vi "new.vi"(8 "error in (no error)":errorcluster, 11 "description":string) -> (0 "error out":errorcluster, 3 "ExampleTask_StopNotifier out":refnum<class "Task_BoolStopNotifier.lvclass">)   [LabVIEW 2023, in "Task_BoolStopNotifier.lvclass"]
doc: "Constructor"
uses:
  Task_BoolStopNotifier.lvclass
  Task_BoolStopNotifier.lvclass/Task_BoolStopNotifier.ctl
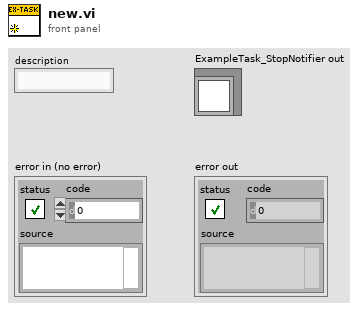
[diagram p1: front panel]
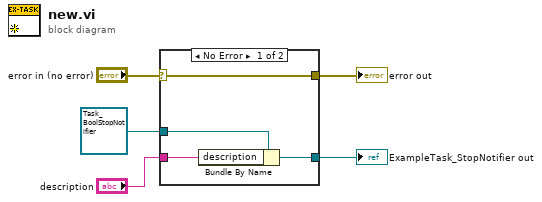
[diagram p0: block diagram]
diagram:
  n1 = case shown="No Error" "error in (no error)" {
    selector: "error in (no error)" -> [w9 w11]
    tunnel: [w9 w11] -> w4
    tunnel: [w8 w10] -> w2
    tunnel: refnum<class "Task_BoolStopNotifier.lvclass"> refnum ("ExampleTask_StopNotifier in") -> [w7 w10]
    tunnel: "description" -> [w6 _]
    frame No Error {
      n2 = Bundle By Name(cluster=w7, "description"=w6) -> (w8:refnum<class "Task_BoolStopNotifier.lvclass">)
    }
    frame Error {
    }
  }
  "error out" <- w4
  "ExampleTask_StopNotifier out" <- w2
